vi "Cache.vi"(7 "Action":T1, 8 "error in (no error)":errorcluster, 10 "VI in":variant, 11 "Thread Name":string) -> (0 "error out":errorcluster, 1 "Found?":bool, 2 "VI out":variant, 3 "Generic VI out":refnum<vi>, 5 "Thread Names":string[](array[string]))   [LabVIEW 2021, in "Thread.lvlib"]
uses:
  Thread.lvlib
  Cache Action.ctl
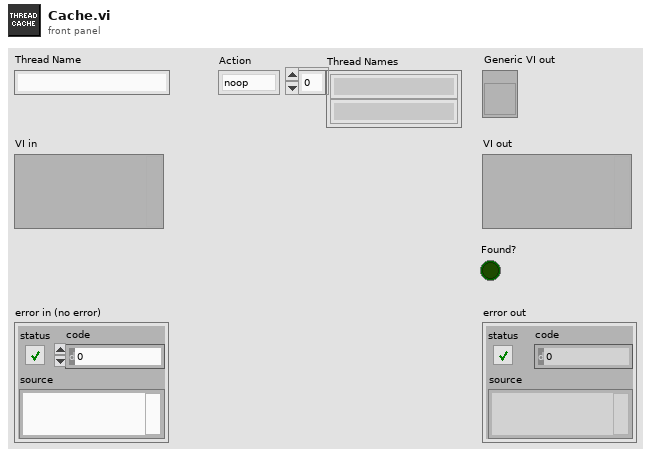
[diagram p1: front panel]
types:
  T1 = typedef "Thread.lvlib/Cache Action.ctl" = enum8{"noop", "get", "add", "remove", "remove_by_ref"}
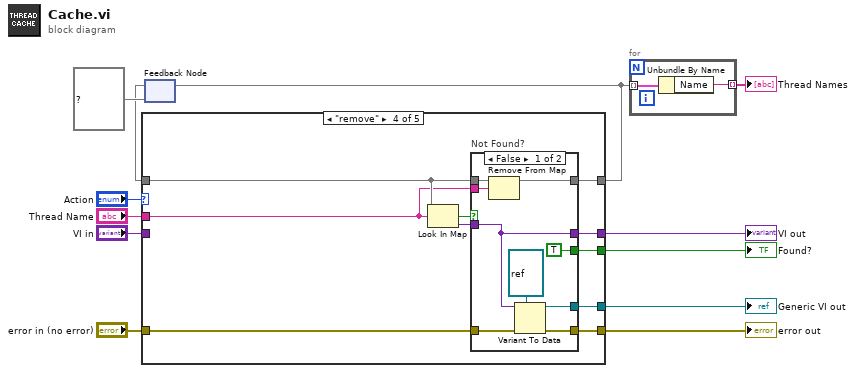
[diagram p0: block diagram]
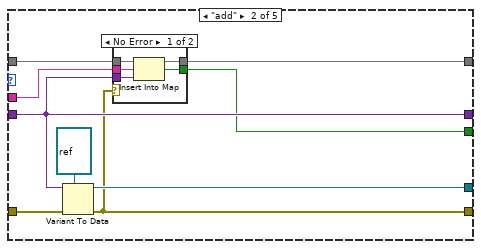
[diagram p3: hidden frame]
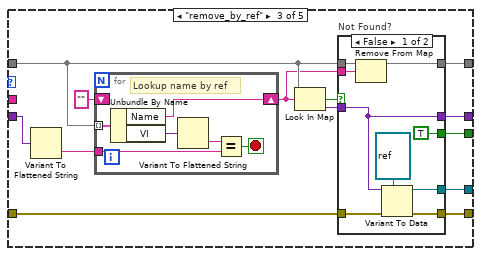
[diagram p5: hidden frame]
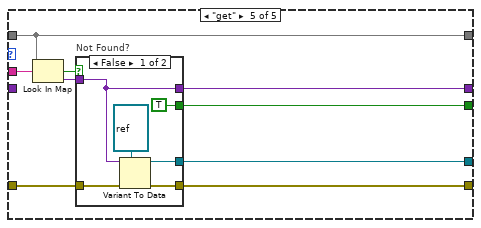
[diagram p8: hidden frame]
diagram:
  n1 = feedback #1(map{string, variant} {} ("Map")) -> (w8:map{string, variant})
  n2 = case shown="\"remove\"" "Action" {
    tunnel: [w13 w15 w41 w68 w88] -> w9
    tunnel: "error in (no error)" -> [w13 w23 w42 w69 w89]
    tunnel: [w14 w21 w39 w66 w81] -> w3
    tunnel: w8 -> [w14 w22 w33 w61 w81]
    tunnel: "Thread Name" -> [_ w20 _ w60 w86]
    tunnel: "VI in" -> [_ w19 w34 _ _]
    tunnel: [_ w19 w36 w63 w83] -> w5
    tunnel: [_ w17 w40 w67 w87] -> w4
    tunnel: [_ w16 w35 w62 w82] -> w1
    frame "noop" {
    }
    frame "add" {
      n3 = Variant To Data(error in=w23, type=refnum<vi> refnum ("Generic VI out"), Variant=w19) -> (data=w17:refnum<vi>, error out=w15:errorcluster)
      n4 = case shown="No Error" w15 {
        tunnel: w22 -> [w28 w29]
        tunnel: [w27 w29] -> w21
        tunnel: w20 -> [w26 _]
        tunnel: w19 -> [w25 _]
        tunnel: [w24 _] -> w16
        frame No Error {
          n5 = Insert Into Map(map in=w28, key=w26, value=w25) -> (map out=w27:map{string, variant}, key already included?=w24:bool)  [unwired: 1 out]
        }
        frame Error {
        }
      }
    }
    frame "remove_by_ref" {
      n6 = Variant To Flattened String(Variant=w34) -> (data string=w31:string)  [unwired: 1 out]
      n7 = for {
        tunnel: w33 -> [w48] mode=indexing
        shift-right: [w46] -> w30
        shift-left: "" ("Name") -> [_]
        tunnel: w31 -> [w44]
        stop <- w43 stop-if-true
        # "Lookup name by ref"
        n8 = Unbundle By Name(w48) -> ("Name"=w46:string, "VI"=w47:variant)
        n9 = Variant To Flattened String(Variant=w47) -> (data string=w45:string)  [unwired: 1 out]
        n10 = Equal?(x=w45, y=w44) -> (x = y?=w43:bool)
      }
      n11 = Look In Map(map=w33, key=w30) -> (key not found?=w37:bool, value=w38:variant)  [unwired: 1 in]
      n12 = case "Not Found?" shown="False" w37 {
        tunnel: w42 -> [w57 w58]
        tunnel: [w56 w58] -> w41
        tunnel: [w54 _] -> w40
        tunnel: w33 -> [w53 w59]
        tunnel: [w52 w59] -> w39
        tunnel: w30 -> [w51 _]
        tunnel: w38 -> [w50 _]
        tunnel: [w50 _] -> w36
        tunnel: [TRUE _] -> w35
        frame False {
          n13 = Remove From Map(10:w51, 11:w53) -> (3:w52:map{string, variant})  [unwired: 2 out]
          n14 = Variant To Data(error in=w57, type=refnum<vi> refnum ("Generic VI out"), Variant=w50) -> (data=w54:refnum<vi>, error out=w56:errorcluster)
        }
        frame True {
        }
      }
    }
    frame "remove" {
      n15 = Look In Map(map=w61, key=w60) -> (key not found?=w64:bool, value=w65:variant)  [unwired: 1 in]
      n16 = case "Not Found?" shown="False" w64 {
        tunnel: w69 -> [w78 w79]
        tunnel: [w77 w79] -> w68
        tunnel: [w75 _] -> w67
        tunnel: w61 -> [w74 w80]
        tunnel: [w73 w80] -> w66
        tunnel: w60 -> [w72 _]
        tunnel: w65 -> [w71 _]
        tunnel: [w71 _] -> w63
        tunnel: [TRUE _] -> w62
        frame False {
          n17 = Remove From Map(10:w72, 11:w74) -> (3:w73:map{string, variant})  [unwired: 2 out]
          n18 = Variant To Data(error in=w78, type=refnum<vi> refnum ("Generic VI out"), Variant=w71) -> (data=w75:refnum<vi>, error out=w77:errorcluster)
        }
        frame True {
        }
      }
    }
    frame "get" {
      n19 = Look In Map(map=w81, key=w86) -> (key not found?=w84:bool, value=w85:variant)  [unwired: 1 in]
      n20 = case "Not Found?" shown="False" w84 {
        tunnel: w89 -> [w95 w96]
        tunnel: [w94 w96] -> w88
        tunnel: [w92 _] -> w87
        tunnel: w85 -> [w91 _]
        tunnel: [w91 _] -> w83
        tunnel: [TRUE _] -> w82
        frame False {
          n21 = Variant To Data(error in=w95, type=refnum<vi> refnum ("Generic VI out"), Variant=w91) -> (data=w92:refnum<vi>, error out=w94:errorcluster)
        }
        frame True {
        }
      }
    }
  }
  "error out" <- w9
  "Generic VI out" <- w4
  "VI out" <- w5
  "Found?" <- w1
  n22 = feedback-in #1(w3) -> ()
  n23 = for {
    tunnel: w3 -> [w98] mode=indexing
    tunnel: [w97] -> w2 mode=indexing
    n24 = Unbundle By Name(w98) -> ("Name"=w97:string)
  }
  "Thread Names" <- w2
